vi "Manual_Cool_Heat_V2.vi"(8 "error in":errorcluster, 11 "DataCluster":T1={"Core"={"Current VI Reference"=refnum, "Close Panel on Exit?"=FALSE, "Exit"=FALSE, "Initialized?"=FALSE}, "Connections"={"cDAQ"={"Task"="", "Connected"=FALSE, "Active"=FALSE, "ID"=""}, "Camera"={"Session"="", "Connected"=FALSE, "Active"=FALSE, "Placeholder"=refnum}, "PSU"={"Port"="", "Connected"=FALSE, "Active"=FALSE}, "Arduino"={"Port"="", "Connected"=FALSE, "Active"=FALSE}}, "Data Acquisition"={"Setup"={"Label"="", "Operator"="", "Notes"="", "TempGrad"=0.0, "TargetTemp"=0.0, "Sample Volume"=1.0}, "Camera"={"Image"=refnum, "Save Image"=refnum, "Image Frequency"=20, "Rectangle"={"Left"=0, "Top"=0, "Right"=0, "Bottom"=0, "Rotation"=0.0}, "Calibration"={"Top Left"={"X"=0.0, "Y"=0.0}, "Top Right"={"X"=0.0, "Y"=0.0}, "Bottom Left"={"X"=0.0, "Y"=0.0}, "Bottom Right"={"X"=0.0, "Y"=0.0}, "Fixpoint"={"X"=0.0, "Y"=0.0}, "Scan Area"=0.0, "Fixpoint Area"=0.0, "Well Pixels"=[], "Valid"=FALSE}, "FocusPos"=0, "Display Mapping"=10, "Camera Mode"=10}, "Thermistor"={"Sample Size"=0, "Calibration"={"B0.100"=[], "R25"=[], "c"=[], "State"=[], "V_S"=0.0, "R_S"=0.0}, "Timing Mode"=14713}, "Partition"={"Data"=[], "Cell Label"="", "Cell Color"=0, "Height"=10, "Width"=16, "Grid"=[]}, "Queue"={"Size"=0, "Queue"=refnum}, "Sample Rate"=0, "Active"=FALSE, "Ready"=FALSE, "Graph Mode"=0, "Gradient Buffer"=2}, "Control"={"Sample Rate"=0, "PID gains"={"proportional gain (Kc)"=0.0, "integral time (Ti, min)"=0.0, "derivative time (Td, min)"=0.0}}, "Manual Temp Control"={"TargetTemp"=1.0, "Mode"=0, "Active"=FALSE}} {"Manual Temp Control"."Mode" items=["Cool", "Heat"]; "Manual Temp Control"."TargetTemp" min=-40.0 max=40.0 step=0.5 format="%#_g °C"; "Control"."PID gains"."derivative time (Td, min)" format="%.3f"; "Control"."PID gains"."integral time (Ti, min)" format="%.3f"; "Control"."PID gains"."proportional gain (Kc)" format="%.3f"; "Control"."Sample Rate" min=1 max=20 step=1 format="%.0f Samples/sec"; "Data Acquisition"."Gradient Buffer" min=2 max=30 step=1; "Data Acquisition"."Graph Mode" items=["Thermistor Temperature", "Camera Temperature"]; "Data Acquisition"."Thermistor"."Timing Mode" items=["Automatic"=16097, "High Resolution"=10195, "High Speed"=14712, "Best 50 Hz Rejection"=14713, "Best 60 Hz Rejection"=14714, "Custom"=10137]; "Data Acquisition"."Thermistor"."Calibration"."R_S" min=0.1 max=1000.0 format="%#_g kOhm"; "Data Acquisition"."Thermistor"."Calibration"."V_S" min=5.0 max=48.0 format="%#_g V"; "Data Acquisition"."Thermistor"."Calibration"."R25" min=0.1 max=1000.0 format="%#_g kOhm"; "Data Acquisition"."Thermistor"."Calibration"."B0.100" min=100.0 max=10000.0 format="%#_g K"; "Data Acquisition"."Thermistor"."Sample Size" min=1 max=200; "Data Acquisition"."Sample Rate" min=20 max=240 format="%.0f samples/min"; "Data Acquisition"."Queue"."Size" min=1 max=200; "Data Acquisition"."Camera"."Camera Mode" items=["Temperature Linear", "Signal Linear"]; "Data Acquisition"."Camera"."Display Mapping" items=["Default"=10, "Most Significant Bits"=11, "Full Dynamic"=12, "Downshift"=13, "Given Range"=14, "90% Dynamic"=15, "Given Percent Range"=16]; "Data Acquisition"."Camera"."Calibration"."Fixpoint"."Y" format="%.2f"; "Data Acquisition"."Camera"."Calibration"."Fixpoint"."X" format="%.2f"; "Data Acquisition"."Camera"."Calibration"."Top Left"."Y" format="%.2f"; "Data Acquisition"."Camera"."Calibration"."Top Left"."X" format="%.2f"; "Data Acquisition"."Camera"."Calibration"."Top Right"."Y" format="%.2f"; "Data Acquisition"."Camera"."Calibration"."Top Right"."X" format="%.2f"; "Data Acquisition"."Camera"."Calibration"."Bottom Left"."Y" format="%.2f"; "Data Acquisition"."Camera"."Calibration"."Bottom Left"."X" format="%.2f"; "Data Acquisition"."Camera"."Calibration"."Bottom Right"."Y" format="%.2f"; "Data Acquisition"."Camera"."Calibration"."Bottom Right"."X" format="%.2f"; "Data Acquisition"."Camera"."Rectangle"."Rotation" min=-90.0 max=90.0 step=1.0 format="%.2f"; "Data Acquisition"."Camera"."Rectangle"."Left" scale=0.0..1024.0; "Data Acquisition"."Camera"."Rectangle"."Right" scale=0.0..1024.0; "Data Acquisition"."Camera"."Image Frequency" min=1 max=60 step=1; "Data Acquisition"."Setup"."Sample Volume" min=0.0 max=500.0 format="%#_g µL"; "Data Acquisition"."Setup"."TargetTemp" min=-40.0 max=40.0 step=0.5 format="%#_g °C"; "Data Acquisition"."Setup"."TempGrad" min=-100.0 max=100.0 step=0.1 format="%#_g °C/min"}) -> (0 "error out":errorcluster)   [LabVIEW 2022 SP3]
uses:
  DataCluster.ctl
  <vilib>/userdefined/High Color/IMAQdx.ctl
  <vilib>/vision/Image Controls.llb/IMAQ Image.ctl
  <vilib>/Platform/TimedLoop/XDataNode/timing_clust.ctl
  <vilib>/Platform/TimedLoop/XDataNode/nitl_modes.ctl
  <vilib>/Platform/TimedLoop/XDataNode/wakeup.ctl
  <extravilib>/ChannelInstances/Stream-bool/Read With Abort.vi
  <extravilib>/ChannelInstances/Tag-c(c(ref(LVObjVI()),bool),bool,bool,u32[Cool,Heat])/Write With Abort.vi
  <extravilib>/ChannelInstances/Tag-bool/Write With Abort.vi
  <extravilib>/ChannelInstances/Tag-bool/Read With Abort.vi
  <extravilib>/ChannelInstances/Tag-c(c(ref(LVObjVI()),bool),bool,bool,u32[Cool,Heat])/Read With Abort.vi
  <extravilib>/ChannelInstances/Stream-bool/Write With Abort.vi
  <extravilib>/ChannelInstances/Stream-bool/EndpointRead.vi
  <extravilib>/ChannelInstances/Stream-bool/Endpoint.vi
  <extravilib>/ChannelInstances/Tag-c(c(ref(LVObjVI()),bool),bool,bool,u32[Cool,Heat])/Instantiate.vi
  <extravilib>/ChannelInstances/Tag-bool/Instantiate.vi
  <extravilib>/ChannelInstances/Stream-bool/Instantiate.vi
  <extravilib>/ChannelInstances/Stream-bool/)Channel.vi
  <resource>/ChannelSupport/_ChannelSupport/WaitIfNeeded.vi
  <extravilib>/ChannelInstances/Tag-c(c(ref(LVObjVI()),bool),bool,bool,u32[Cool,Heat])/Endpoint.vi
  <extravilib>/ChannelInstances/Tag-bool/Endpoint.vi
  <extravilib>/ChannelInstances/Tag-bool/EndpointRead.vi
  <extravilib>/ChannelInstances/Tag-c(c(ref(LVObjVI()),bool),bool,bool,u32[Cool,Heat])/EndpointRead.vi
  <vilib>/platform/TimedLoop/XDataNode/XDataNode.xnode
  <vilib>/Platform/TimedLoop/XDataNode/XDNodeRunTimeDep.lvlib
  <extravilib>/ChannelInstances/Tag-bool.lvlib
  <extravilib>/ChannelInstances/Stream-bool.lvlib
  <extravilib>/ChannelInstances/Tag-c(c(ref(LVObjVI()),bool),bool,bool,u32[Cool,Heat]).lvlib
panel:
  in  "Cool/Heat":enum32{"Cool", "Heat"}(ring)
  in  "Start":bool
  in  "OK":bool
  in  "Intensisty":i32(slide)=50 min=0 max=100 step=10 scale=0.0..100.0 scale format="%.0f %%"
  out "Manual":waveform(dbl)[](graph)=[{"t0"=timestamp(0 s since 1904-01-01), "dt"=0.5, "Y"=[-0.5459297948238789, -0.5384662523625495, -0.5305055716687722, -0.5227516337304128, -0.5152151485633342, -0.5074594731778411, -0.5000110550794236, -0.49229613528221505, -0.48455544270581347, -0.47704875214651904, -0.4694184221817747, -0.4617297562684411, -0.4542538363910736, -0.44666324774779786, -0.43914993037163397, -0.4315969934450372, -0.42413652957329057, -0.41648702187743, -0.4090503718449979, -0.40158637492342547, -0.3941665018638969, -0.38661414017374235, -0.3792972035366138, -0.37178469009330656, -0.3640722423599955, -0.3568479440776631, -0.3495051306403334, -0.3421642645601655, -0.33493653098477, -0.3275193397439705, -0.32018295336060504, -0.3128894600430486, -0.3055440591103306, -0.29873448073929, -0.29143683883588484, -0.2843423086450982, -0.2772355209388995, -0.27008916517709947, -0.26279625635638254, -0.2557072429162988, -0.24884447893036513, -0.2418962610460262, -0.23471006933283486, -0.22766777081987025, -0.22069024864064335, -0.21390317409486895, -0.20710909597313554, -0.20017922598796378, -0.19328186072145903, -0.18648965958030286, -0.17982101574808698, -0.17308125272085514, -0.16650153019624944, -0.15972005812583243, -0.15288052381799008, -0.14672994680516058, -0.14007374846858675, -0.1336178193214643, -0.12705690492929214, -0.12060549031730709, -0.11444511771368156, -0.10804984536035589, -0.10172786836292154, -0.09532872836465985, -0.08927381125350682, -0.08296971036909855, -0.07689207711853907, -0.07078036829076739, -0.06468688490901309, -0.058868939175738766, -0.05270999822746214, -0.04685361027102993, -0.04104637566433278]}, {"t0"=timestamp(0 s since 1904-01-01), "dt"=0.5, "Y"=[-30.0, -30.0, -30.0, -30.0, -30.0, -30.0, -30.0, -30.0, -30.0, -30.0, -30.0, -30.0, -30.0, -30.0, -30.0, -30.0, -30.0, -30.0, -30.0, -30.0, -30.0, -30.0, -30.0, -30.0, -30.0, -30.0, -30.0, -30.0, -30.0, -30.0, -30.0, -30.0, -30.0, -30.0, -30.0, -30.0, -30.0, -30.0, -30.0, -30.0, -30.0, -30.0, -30.0, -30.0, -30.0, -30.0, -30.0, -30.0, -30.0, -30.0, -30.0, -30.0, -30.0, -30.0, -30.0, -30.0, -30.0, -30.0, -30.0, -30.0, -30.0, -30.0, -30.0, -30.0, -30.0, -30.0, -30.0, -30.0, -30.0, -30.0, -30.0, -30.0, -30.0]}]
  out "Status":string="System ready"
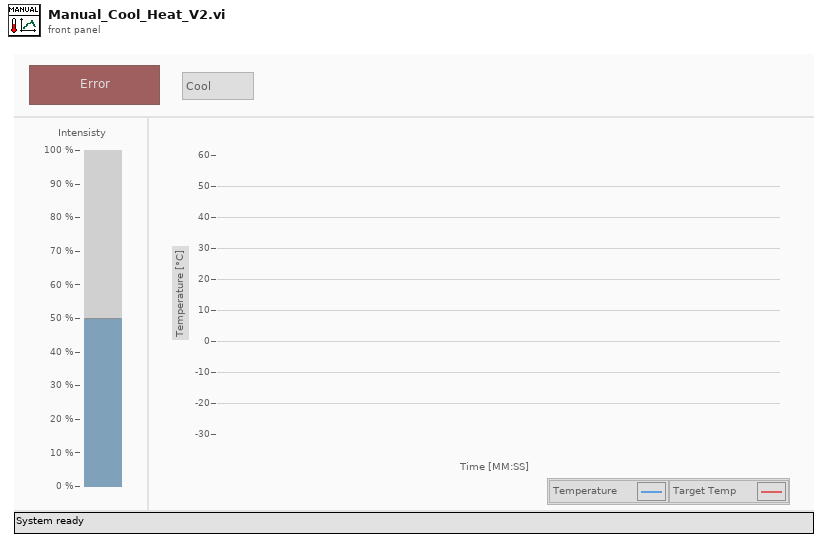
[diagram p1: front panel]
types:
  T1 = typedef "DataCluster.ctl" = cluster{"Core":cluster{"Current VI Reference":refnum<vi>, "Close Panel on Exit?":bool, "Exit":bool, "Initialized?":bool}, "Connections":cluster{"cDAQ":cluster{"Task":refnum<k21>, "Connected":bool, "Active":bool, "ID":string}, "Camera":cluster{"Session":T2, "Connected":bool, "Active":bool, "Placeholder":T3}, "PSU":cluster{"Port":refnum<visa-resource-name>, "Connected":bool, "Active":bool}, "Arduino":cluster{"Port":refnum<visa-resource-name>, "Connected":bool, "Active":bool}}, "Data Acquisition":cluster{"Setup":cluster{"Label":string, "Operator":string, "Notes":string, "TempGrad":dbl, "TargetTemp":dbl, "Sample Volume":dbl}, "Camera":cluster{"Image":T3, "Save Image":T3, "Image Frequency":i32, "Rectangle":T4, "Calibration":cluster{"Top Left":T5, "Top Right":T5, "Bottom Left":T5, "Bottom Right":T5, "Fixpoint":T5, "Scan Area":dbl, "Fixpoint Area":dbl, "Well Pixels":cluster{"X":i32, "Y":i32}[][], "Valid":bool}, "FocusPos":u32, "Display Mapping":u32, "Camera Mode":u32}, "Thermistor":cluster{"Sample Size":i32, "Calibration":cluster{"B0.100":dbl[], "R25":dbl[], "c":dbl[][], "State":bool[], "V_S":dbl, "R_S":dbl}, "Timing Mode":i32}, "Partition":cluster{"Data":string[][], "Cell Label":string, "Cell Color":u32, "Height":i32, "Width":i32, "Grid":string[][]}, "Queue":cluster{"Size":i32, "Queue":refnum<queue>}, "Sample Rate":i32, "Active":bool, "Ready":bool, "Graph Mode":u16, "Gradient Buffer":i32}, "Control":cluster{"Sample Rate":i32, "PID gains":cluster{"proportional gain (Kc)":dbl, "integral time (Ti, min)":dbl, "derivative time (Td, min)":dbl}}, "Manual Temp Control":cluster{"TargetTemp":dbl, "Mode":u16, "Active":bool}}
  T2 = typedef "IMAQdx.ctl" = refnum<k21>
  T3 = typedef "IMAQ Image.ctl" = refnum<image>
  T4 = typedef "IMAQ Rectangle" = cluster{"Left":i32, "Top":i32, "Right":i32, "Bottom":i32, "Rotation":dbl}
  T5 = typedef "IMAQ Point" = cluster{"X":sgl, "Y":sgl}
  T6 = enum8{"Enabled", "Disabled", "Disabled and Grayed Out"}
  T7 = enum32{"Invalid", "Standard", "Closed", "Hidden", "Minimized", "Maximized"}
  T8 = enum32{"invalid app kind", "Development System", "Run Time System", "Student Edition", "Embedded LabVIEW", "Evaluation", "Custom"}
  T9 = cluster{"Core":cluster{"Current VI Reference":refnum<vi>, "Close Panel on Exit?":bool}, "Active":bool, "Ready":bool, "Cool/Heat":enum32{"Cool", "Heat"}}
  T10 = cluster{"Current VI Reference":refnum<vi>, "Close Panel on Exit?":bool}
  T11 = typedef "Tag-bool.lvlib/))Channel.ctl" = refnum<queue>
  T12 = typedef "Tag-c(c(ref(LVObjVI()),bool),bool,bool,u32[Cool,Heat]).lvlib/))Channel.ctl" = refnum<queue>
  T13 = typedef "XDNodeRunTimeDep.lvlib/timing_clust.ctl" = cluster{"Expected End [f-1]":u64, "Actual End [f-1]":u64, "Finished Late? [f-1]":bool, "Expected End [i-1]":u64, "Actual End [i-1]":u64, "Finished Late? [i-1]":bool, "Expected Start [i]":u64, "Actual Start [i]":u64, "Expected Start [f]":u64, "Actual Start [f]":u64, "Source Name":string, "Structure Name":string, "Period":i64, "Deadline":i64, "Offset":i64, "Start":i64, "Priority":i32, "Timeout":i32, "Mode":T14, "Wakeup Reason":T15, "Error":errorcluster, "Source Type":string, "Secondary Source Type":string, "Global End Time":u64, "Global Start Time":u64, "Frame Duration":u64, "Iteration Duration":u64, "Assigned CPU":i32, "I/O Scan Engine Mode":u32}
  T14 = typedef "XDNodeRunTimeDep.lvlib/nitl_modes.ctl" = enum32{"No Change", "Process missed periods, maintain original phase", "Discard missed periods, maintain original phase", "Process missed periods, ignore original phase", "Discard missed periods, ignore original phase"}
  T15 = typedef "XDNodeRunTimeDep.lvlib/wakeup.ctl" = enum32{"Normal", "Aborted", "Asynchronous wakeup", "Timing source error", "Timed loop error", "Timeout"}
  T16 = typedef "Stream-bool.lvlib/)Channel.ctl" = refnum<queue>
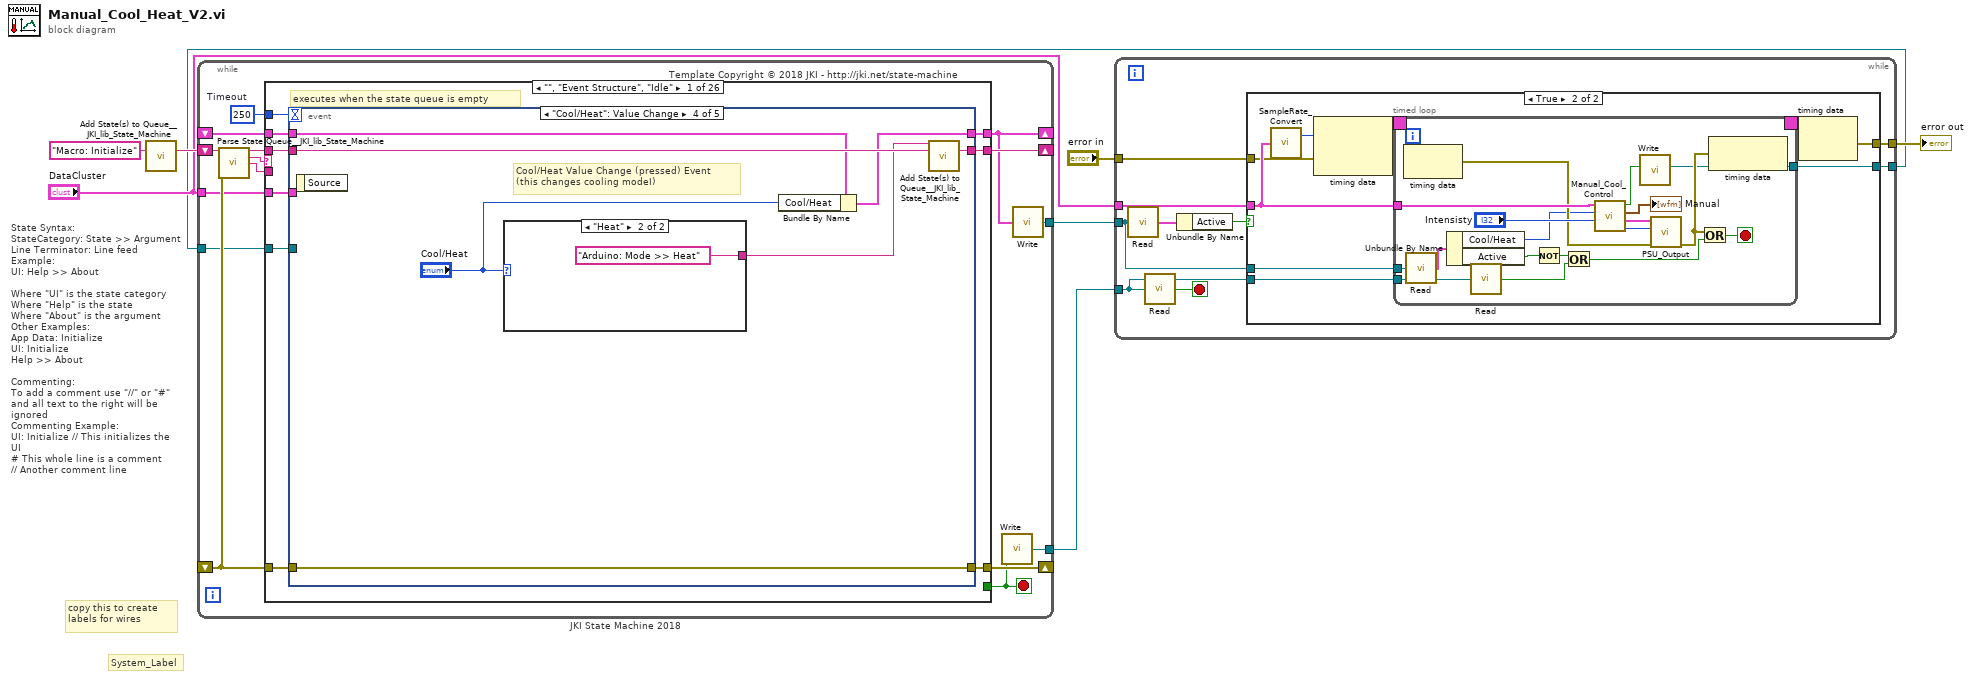
[diagram p0: block diagram]
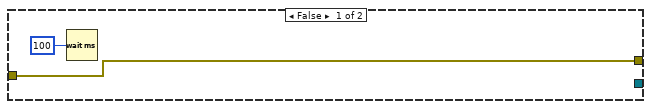
[diagram p2: hidden frame]
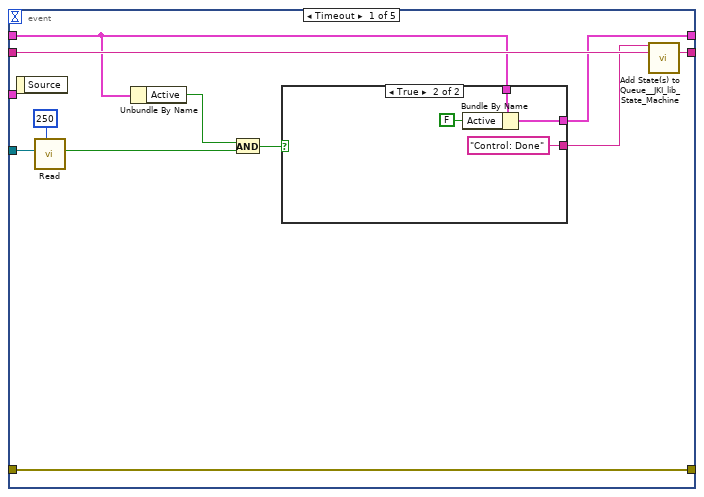
[diagram p3: hidden frame]
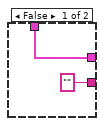
[diagram p4: hidden frame]
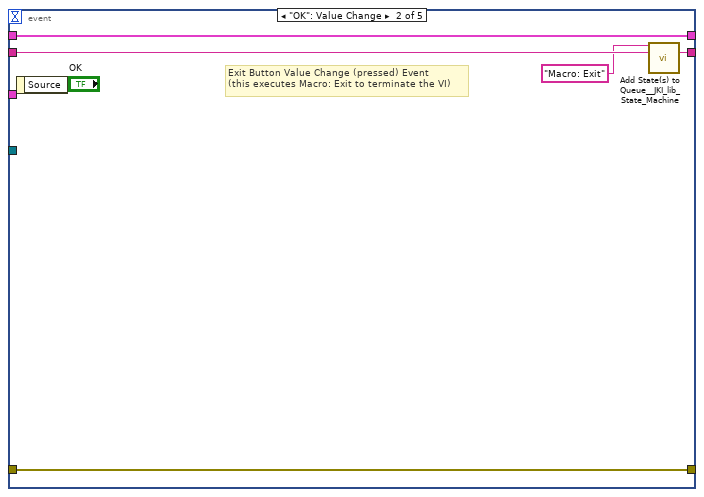
[diagram p5: hidden frame]
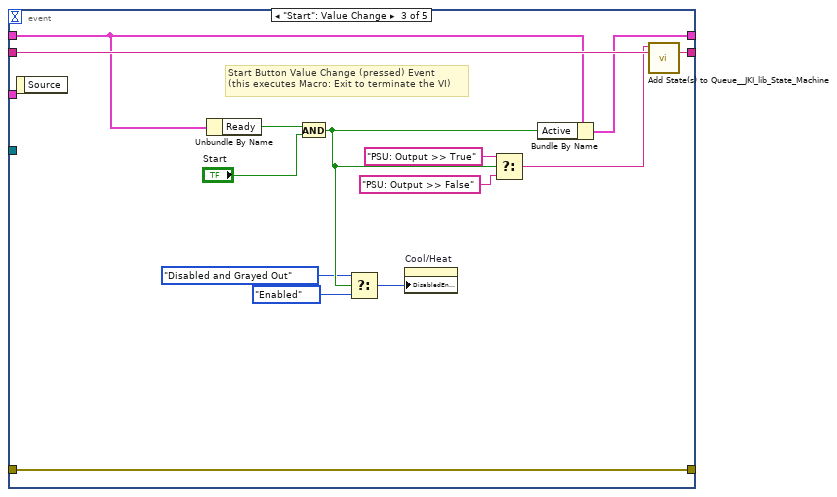
[diagram p6: hidden frame]
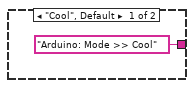
[diagram p7: hidden frame]
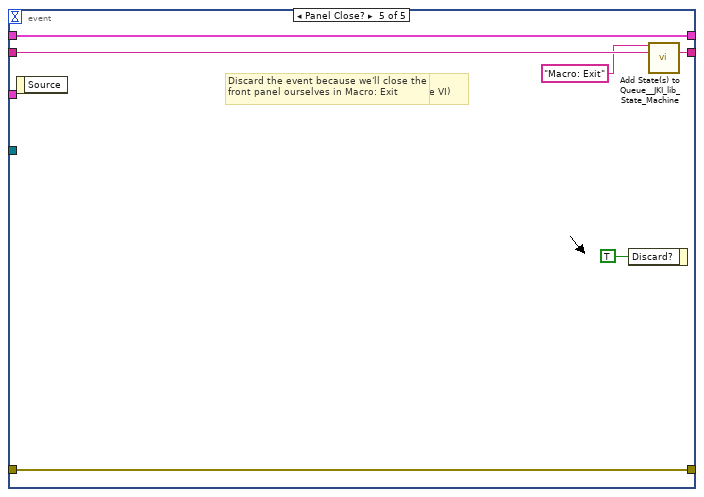
[diagram p8: hidden frame]
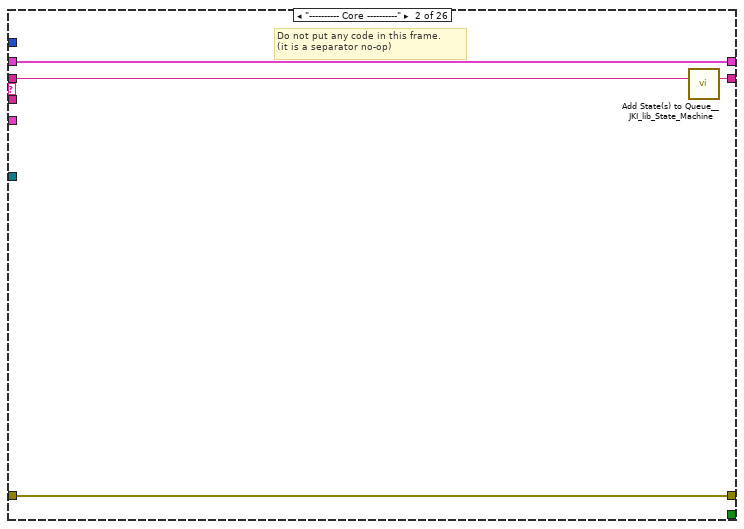
[diagram p9: hidden frame]
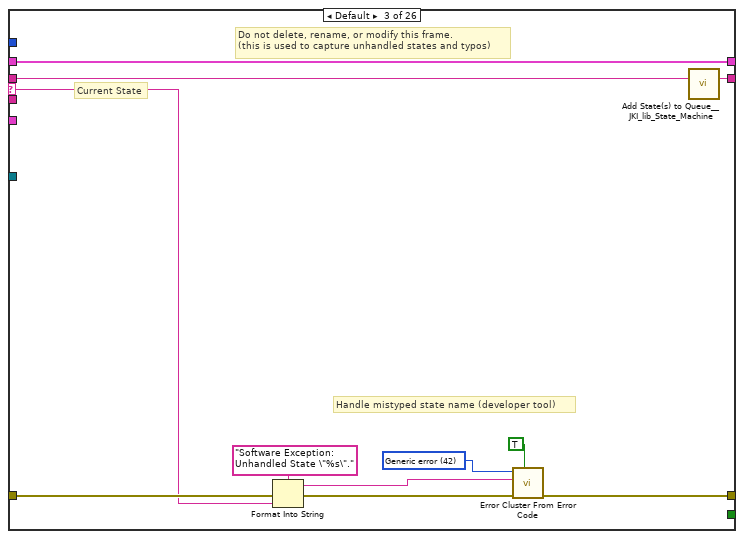
[diagram p10: hidden frame]
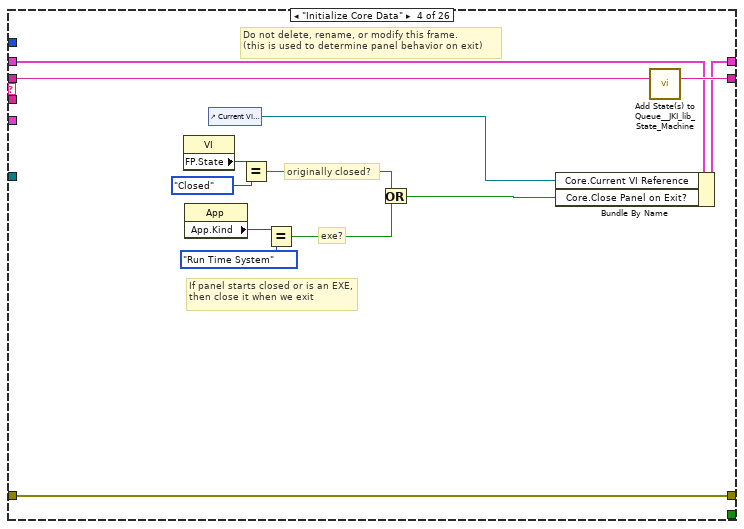
[diagram p11: hidden frame]
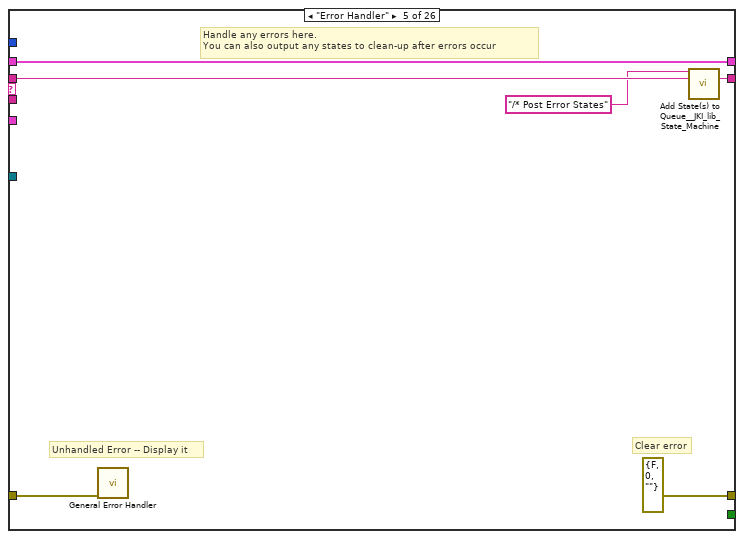
[diagram p12: hidden frame]
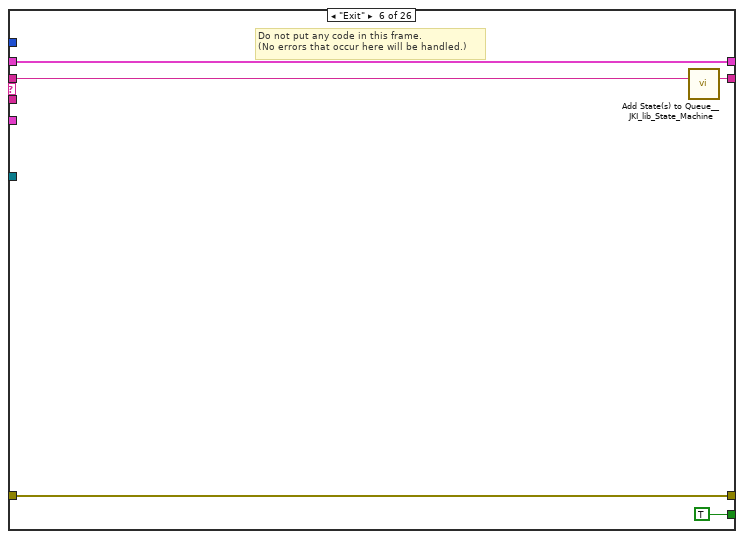
[diagram p13: hidden frame]
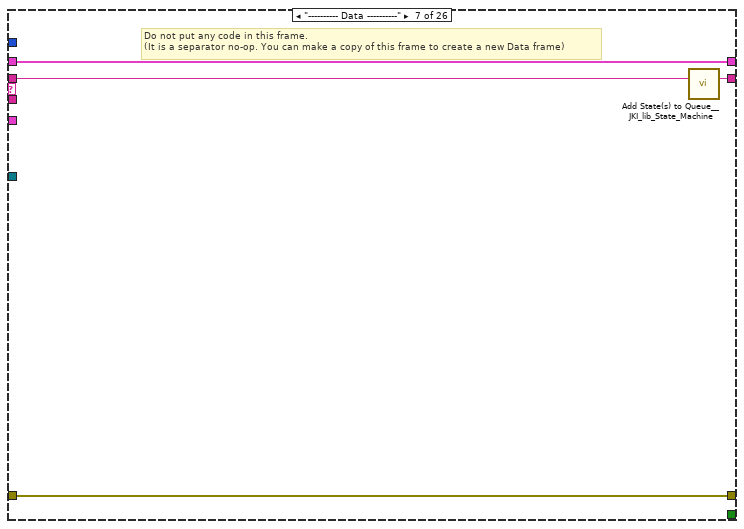
[diagram p14: hidden frame]
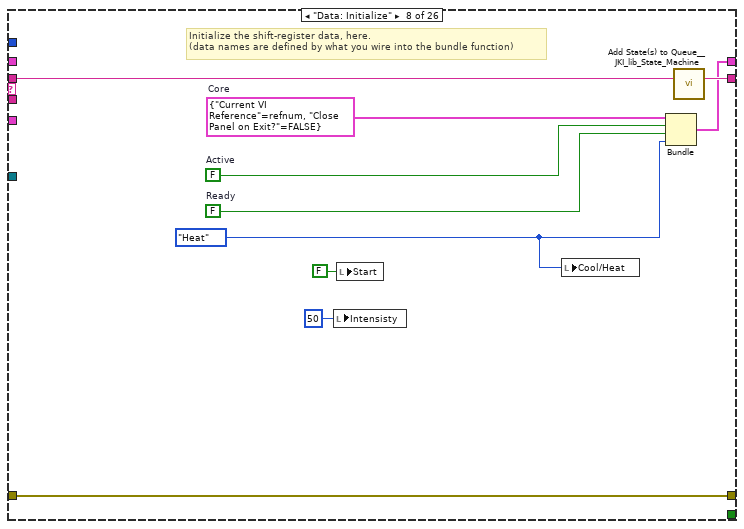
[diagram p15: hidden frame]
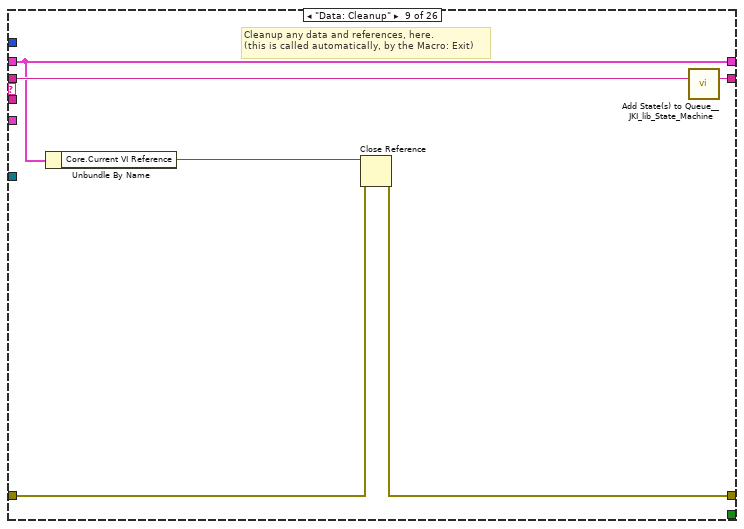
[diagram p16: hidden frame]
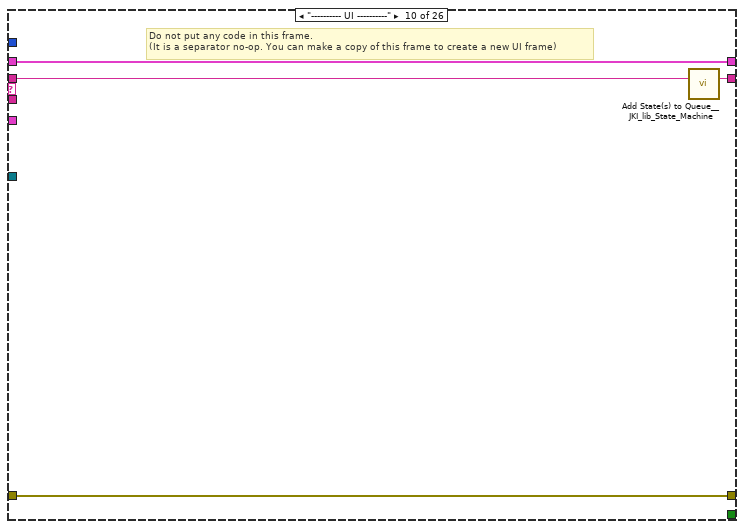
[diagram p17: hidden frame]
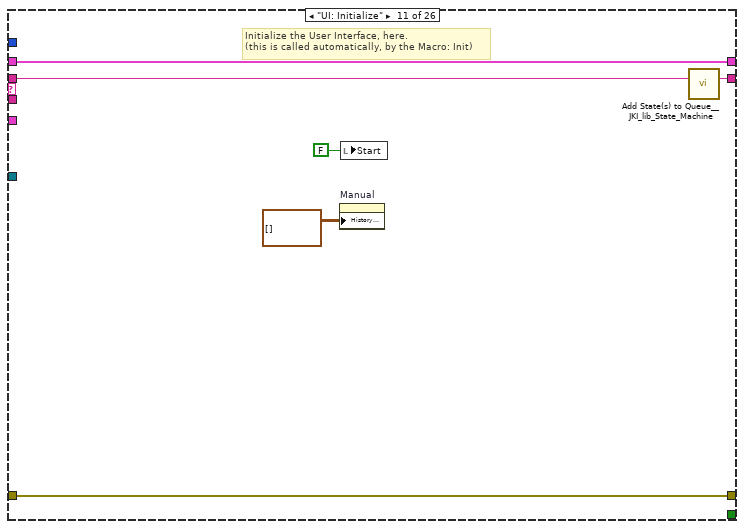
[diagram p18: hidden frame]
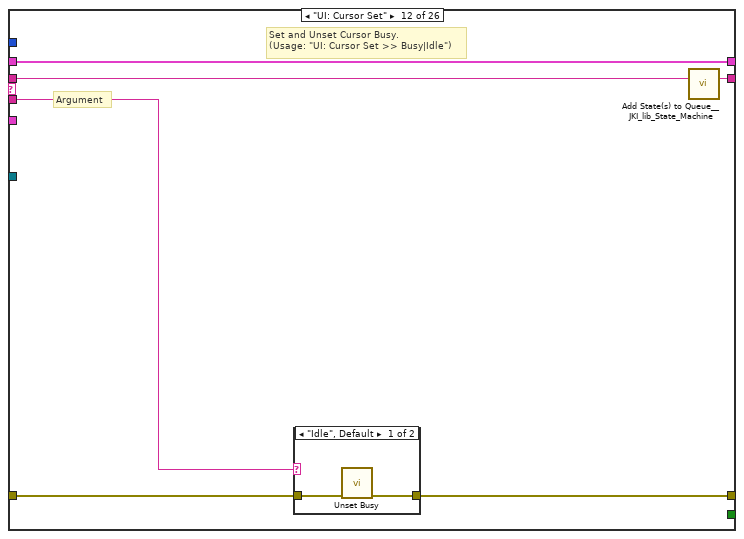
[diagram p19: hidden frame]
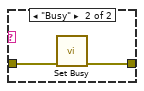
[diagram p20: hidden frame]
diagram:
  # "State Syntax:\nStateCategory: State >> Argument\nLine Terminator: Line feed\nExample:\nUI: Help >> About\n\nWhere \"UI\" is the state category\nWhere \"Help\" is the state\nWhere \"About\" is the argument\nOther Examples:\nApp Data: Initialize\nUI: Initialize\nHelp >> About\n\nCommenting:\nTo add a comment use \"//\" or \"#\" and all text to the right will be ignored\nCommenting Example:\nUI: Initialize // This initializes the UI\n# This whole line is a comment\n// Another comment line"
  # "copy this to create labels for wires"
  # "System_Label"
  n1 = call <vilib>:"Add State(s) to Queue__JKI_lib_State_Machine.vi"("State(s) in (\"\")"="Macro: Initialize") -> ("States Out"=w8:string)  [unwired: 14 in]
  n2 = while "JKI State Machine 2018" {
    shift-right: [w16] -> _
    shift-left: _ -> [w15]
    shift-right: [w19] -> _
    shift-left: _ -> [w13]
    shift-right: [w18] -> _
    shift-left: w8 -> [w20]
    tunnel: "DataCluster" -> [w12]
    tunnel: w3 -> [w11]
    tunnel: [w10] -> w2
    tunnel: [w9] -> w1
    stop <- w17 stop-if-true
    w14 = 250  # Timeout
    # "Template Copyright © 2018 JKI - http://jki.net/state-machine"
    n3 = call <vilib>:"Parse State Queue__JKI_lib_State_Machine.vi"("State Queue"=w20, "Error In (no error)"=w13) -> ("Remaining States"=w22:string, "Current State"=w23:string, "Arguments"=w21:string)  [unwired: 11 in]
    n4 = case shown="\"\", \"Event Structure\", \"Idle\"" w23 {
      selector: w23 -> [_ _ w88 _ _ _ _ _ _ _ _ _ _ _ _ _ _ _ _ _ _ _ _ _ _ _]
      tunnel: w22 -> [w32 w87 w92 w111 w117 w122 w126 w136 w142 w146 w152 w158 w167 w174 w243 w248 w258 w262 w278 w286 w295 w316 w323 w327 w335 w346]
      tunnel: w21 -> [_ _ _ _ _ _ _ _ _ _ _ w153 w163 w168 _ _ _ _ _ _ _ _ _ _ w330 w342]
      tunnel: w15 -> [w30 w84 w90 w104 w114 w120 w123 _ w137 w143 w150 w156 w165 w170 w240 w245 w255 w259 w275 w284 w293 w314 w319 w324 w333 w344]
      tunnel: [w29 w85 w94 w108 errorcluster {"status"=FALSE, "code"=0, "source"=""} ("error out") w119 w124 w133 w138 w144 w149 w154 w164 w171 w241 w246 w256 w260 w276 w283 w292 w313 w321 w325 w328 w341] -> w19
      tunnel: w13 -> [w28 w85 w93 w108 w113 w119 w124 w133 w139 w144 w149 w155 w164 w172 w241 w246 w256 w260 w276 w283 w292 w313 w321 w325 w329 w341]
      tunnel: [w31 w86 w91 w110 w116 w121 w125 w135 w141 w145 w151 w157 w166 w173 w242 w247 w257 w261 w277 w285 w294 w315 w322 w326 w334 w345] -> w18
      tunnel: [_ _ _ _ _ TRUE _ _ _ _ _ _ _ _ _ _ _ _ _ _ _ _ _ _ _ _] -> w17
      tunnel: [w27 w84 w90 w109 w114 w120 w123 w134 w137 w143 w150 w156 w165 w170 w240 w245 w255 w259 w267 w284 w293 w314 w320 w324 w333 w344] -> w16
      tunnel: w14 -> [w26 _ _ _ _ _ _ _ _ _ _ _ _ _ _ _ _ _ _ _ _ _ _ _ _ _]
      tunnel: w12 -> [w25 _ _ _ _ _ _ _ _ _ _ _ _ _ _ _ _ _ w274 _ _ w310 _ _ w331 w343]
      tunnel: w11 -> [w24 _ _ _ _ _ _ _ _ _ _ _ _ _ _ _ _ _ _ _ _ _ _ _ _ _]
      frame "", "Event Structure", "Idle" {
        # "executes when the state queue is empty"
        n5 = event shown="[3] \"Cool/Heat\": Value Change" {
          selector: _ -> [_ _ _ _ _]
          dyn-events: _ -> [_ _ _ _ _]
          timeout: w26 -> [_ _ _ _ _]
          tunnel: w32 -> [w43 w54 w68 w75 w83]
          tunnel: [w42 w53 w67 w74 w82] -> w31
          tunnel: w30 -> [w39 w51 w61 w72 w80]
          tunnel: [w41 w52 w66 w73 w81] -> w29
          tunnel: w28 -> [w41 w52 w66 w73 w81]
          tunnel: [w36 w51 w62 w70 w80] -> w27
          tunnel: w25 -> [_ _ _ _ _]
          tunnel: w24 -> [w40 _ _ _ _]
          event Timeout {
            n6 = event-data() -> ()  [unwired: 1 in, 1 out]
            n7 = call <extravilib>:"Read.vi"("timeout in ms (-1)"=250, "channel"=w40) -> ("element"=w37:bool)  [unwired: 5 in, 4 out]
            n8 = Unbundle By Name(w39) -> ("Active"=w38:bool)
            n9 = And(x=w38, y=w37) -> (x .and. y?=w34:bool)
            n10 = case shown="True" w34 {
              tunnel: w39 -> [w45 w49]
              tunnel: [w45 w48] -> w36
              tunnel: ["" "Control: Done"] -> w33
              frame False {
              }
              frame True {
                n11 = Bundle By Name(cluster=w49, "Active"=FALSE) -> (w48:T9)
              }
            }
            n12 = call <vilib>:"Add State(s) to Queue__JKI_lib_State_Machine.vi"("State(s) in Front (\"\")"=w33, "State(s) in (\"\")"=w43) -> ("States Out"=w42:string)  [unwired: 13 in]
          }
          event "OK": Value Change {
            # "Exit Button Value Change (pressed) Event\n(this executes Macro: Exit to terminate the VI)"
            n13 = event-data() -> ()  [unwired: 1 in, 1 out]
            n14 = call <vilib>:"Add State(s) to Queue__JKI_lib_State_Machine.vi"("State(s) in Front (\"\")"="Macro: Exit", "State(s) in (\"\")"=w54) -> ("States Out"=w53:string)  [unwired: 13 in]
          }
          event "Start": Value Change {
            # "Start Button Value Change (pressed) Event\n(this executes Macro: Exit to terminate the VI)"
            n15 = event-data() -> ()  [unwired: 1 in, 1 out]
            n16 = Unbundle By Name(w61) -> ("Ready"=w60:bool)
            n17 = And(x=w60, y="Start") -> (x .and. y?=w58:bool)
            n18 = Select(t=T6."Disabled and Grayed Out" ("Disabled"), s=w58, f=T6."Enabled" ("Disabled")) -> (s? t:f=w57:T6)
            n19 = property on="Cool/Heat" class="Enum (strict)"("DisabledEnum"=w57) -> ()  [unwired: 2 in, 2 out]
            n20 = Select(t="PSU: Output >> True", s=w58, f="PSU: Output >> False") -> (s? t:f=w63:string)
            n21 = Bundle By Name(cluster=w61, "Active"=w58) -> (w62:T9)
            n22 = call <vilib>:"Add State(s) to Queue__JKI_lib_State_Machine.vi"("State(s) in Front (\"\")"=w63, "State(s) in (\"\")"=w68) -> ("States Out"=w67:string)  [unwired: 13 in]
          }
          event "Cool/Heat": Value Change {
            # "Cool/Heat Value Change (pressed) Event\n(this changes cooling modeI)"
            n23 = event-data() -> ()  [unwired: 1 in, 1 out]
            n24 = case shown="\"Heat\"" "Cool/Heat" {
              tunnel: ["Arduino: Mode >> Cool" "Arduino: Mode >> Heat"] -> w71
              frame "Cool", Default {
              }
              frame "Heat" {
              }
            }
            n25 = Bundle By Name(cluster=w72, "Cool/Heat"="Cool/Heat") -> (w70:T9)
            n26 = call <vilib>:"Add State(s) to Queue__JKI_lib_State_Machine.vi"("State(s) in Front (\"\")"=w71, "State(s) in (\"\")"=w75) -> ("States Out"=w74:string)  [unwired: 13 in]
          }
          event Panel Close? {
            # "Discard the event because we'll close the front panel ourselves in Macro: Exit"
            # "Close Panel button (pressed) Event\n(this executes Macro: Exit to terminate the VI)"
            n27 = event-data() -> ()  [unwired: 1 in, 1 out]
            n28 = event-data("Discard?"=TRUE) -> ()  [unwired: 1 in, 1 out]
            n29 = call <vilib>:"Add State(s) to Queue__JKI_lib_State_Machine.vi"("State(s) in Front (\"\")"="Macro: Exit", "State(s) in (\"\")"=w83) -> ("States Out"=w82:string)  [unwired: 13 in]
          }
        }
      }
      frame "---------- Core ----------" {
        # "Do not put any code in this frame.\n(it is a separator no-op)"
        n30 = call <vilib>:"Add State(s) to Queue__JKI_lib_State_Machine.vi"("State(s) in (\"\")"=w87) -> ("States Out"=w86:string)  [unwired: 14 in]
      }
      frame Default {
        w97 = 42 items=["No error", "Argument error", "Memory is full", "Out of zone", "End of file", "File already open", "Generic file I/O error", "File not found", "File permission error", "Disk is full", "Duplicate path", "Too many files open", "System feature not enabled", "Resource file not found", "Cannot add resource", "Resource not found", "Image not found", "Image memory error", "Pen does not exist", "Config type invalid", "Config token not found", "Config parse error", "Config memory error", "Bad external code format", "Bad external code offset", "External code not present", "Null window", "Destroy window error", "Null menu", "Print aborted", "Bad print record", "Print driver error", "Windows error during printing", "Memory error during printing", "Print dialog error", "Generic print error", "Invalid device refnum", "Device not found", "Device parameter error", "Device unit error", "Cannot open device", "Device call aborted", "Generic error", "Cancelled by user", "Object ID too low", "Object ID too high", "Object not in heap", "Unknown heap", "Unknown object (invalid DefProc)", "Unknown object (DefProc not in table)", "Message out of range", "Invalid (null) method", "Unknown message", "Manager call not supported", "Bad address", "Network operation in progress", "Network operation timed out", "Connection is busy", "Network attribute not supported", "Network error", "Address in use", "System out of memory", "Connection aborted", "Connection refused", "Not connected", "Already connected", "Connection closed", "Initialization error (interapplication manager)", "Bad occurrence", "Wait on unbound occurrence handler", "Occurrence queue overflow", "Datalog type conflict", "Unused", "Unrecognized type (interapplication manager)", "Memory corrupt", "Failed to make temporary DLL", "Old CIN version", "Drag socket not found", "Failed to load drop-object", "Failed to register OLE object", "Failed to release OLE object", "Format specifier type mismatch", "Unknown format specifier", "Too few format specifiers", "Too many format specifiers", "Scan failed", "Newer CIN version", "Error converting to variant", "Runtime menu error", "Password tampered", "Variant attribute not found", "Incompatible variant data type", "Event data is not available", "Event Store is not present", "Occurrence is not found", "Event Queue is not created", "Event info is not available", "Refnum passed is NULL", "Error retrieving Class GUID", "Error retrieving CoClass GUID", "Error retrieving TypeLib GUID.", "Bad built application magic bytes.", "Specific driver is different from the specific driver associated with the Logical Name.", "There is no session opened to the class driver.", "Max Error", "MAX - Error with config objects", "MAX - Error loading configuration", "MAX - Group not supported"]
        # "Current State"
        # "Do not delete, rename, or modify this frame.\n(this is used to capture unhandled states and typos)"
        # "Handle mistyped state name (developer tool)"
        n31 = Format Into String(format string="Software Exception: Unhandled State \"%s\"." ("message"), error in=w93, w88) -> (resulting string=w96:string, error out=w95:errorcluster)  [unwired: 1 in]
        n32 = call <vilib>:"Error Cluster From Error Code.vi"("show call chain? (False)"=TRUE, "error in (no error)"=w95, "error message (\"\")"=w96, "error code (0)"=w97) -> ("error out"=w94:errorcluster)  [unwired: 5 in]
        n33 = call <vilib>:"Add State(s) to Queue__JKI_lib_State_Machine.vi"("State(s) in (\"\")"=w92) -> ("States Out"=w91:string)  [unwired: 14 in]
      }
      frame "Initialize Core Data" {
        # "Do not delete, rename, or modify this frame.\n(this is used to determine panel behavior on exit)"
        # "originally closed?"
        # "exe?"
        # "If panel starts closed or is an EXE, then close it when we exit"
        n34 = property class="VI"() -> ("FP.State"=w101:T7)  [unwired: 2 in, 2 out]
        n35 = property class="App"() -> ("App.Kind"=w107:T8)  [unwired: 2 in, 2 out]
        n36 = control-ref of="Current VI Reference"() -> (w102:refnum<vi>)
        n37 = Equal?(x=w101, y=T7."Closed" ("Front Panel Window:State")) -> (x = y?=w99:bool)
        n38 = Equal?(x=w107, y=T8."Run Time System" ("Application:Kind")) -> (x = y?=w105:bool)
        n39 = Or(x=w99, y=w105) -> (x .or. y?=w103:bool)
        n40 = Bundle By Name(cluster=w104, "Core.Current VI Reference"=w102, "Core.Close Panel on Exit?"=w103) -> (w109:T9)
        n41 = call <vilib>:"Add State(s) to Queue__JKI_lib_State_Machine.vi"("State(s) in (\"\")"=w111) -> ("States Out"=w110:string)  [unwired: 14 in]
      }
      frame "Error Handler" {
        # "Unhandled Error -- Display it"
        # "Handle any errors here.\nYou can also output any states to clean-up after errors occur"
        # "Clear error"
        n42 = call <vilib>:"General Error Handler.vi"("error in (no error)"=w113) -> ()  [unwired: 10 in, 5 out]
        n43 = call <vilib>:"Add State(s) to Queue__JKI_lib_State_Machine.vi"("State(s) in Front (\"\")"="/* Post Error States", "State(s) in (\"\")"=w117) -> ("States Out"=w116:string)  [unwired: 13 in]
      }
      frame "Exit" {
        # "Do not put any code in this frame.\n(No errors that occur here will be handled.)"
        n44 = call <vilib>:"Add State(s) to Queue__JKI_lib_State_Machine.vi"("State(s) in (\"\")"=w122) -> ("States Out"=w121:string)  [unwired: 14 in]
      }
      frame "---------- Data ----------" {
        # "Do not put any code in this frame.\n(It is a separator no-op. You can make a copy of this frame to create a new Data frame)"
        n45 = call <vilib>:"Add State(s) to Queue__JKI_lib_State_Machine.vi"("State(s) in (\"\")"=w126) -> ("States Out"=w125:string)  [unwired: 14 in]
      }
      frame "Data: Initialize" {
        w127 = enum32{"Cool", "Heat"}."Heat" ("Cool/Heat")
        w130 = FALSE  # Ready
        w131 = T10 {"Current VI Reference"=refnum, "Close Panel on Exit?"=FALSE}  # Core
        w132 = FALSE  # Active
        # "Initialize the shift-register data, here.\n(data names are defined by what you wire into the bundle function)"
        n46 = local write "Intensisty"(50 ("Intensisty")) -> ()
        n47 = local write "Start"(FALSE ("Key Focus")) -> ()
        n48 = local write "Cool/Heat"(w127) -> ()
        n49 = Bundle("Core"=w131, "Active"=w132, "Ready"=w130, "Cool/Heat"=w127) -> (w134:T9)  [unwired: 1 in]
        n50 = call <vilib>:"Add State(s) to Queue__JKI_lib_State_Machine.vi"("State(s) in (\"\")"=w136) -> ("States Out"=w135:string)  [unwired: 14 in]
      }
      frame "Data: Cleanup" {
        # "Cleanup any data and references, here.\n(this is called automatically, by the Macro: Exit)"
        n51 = Unbundle By Name(w137) -> ("Core.Current VI Reference"=w140:refnum<vi>)
        n52 = Close Reference(reference=w140, error in (no error)=w139) -> (error out=w138:errorcluster)
        n53 = call <vilib>:"Add State(s) to Queue__JKI_lib_State_Machine.vi"("State(s) in (\"\")"=w142) -> ("States Out"=w141:string)  [unwired: 14 in]
      }
      frame "---------- UI ----------" {
        # "Do not put any code in this frame.\n(It is a separator no-op. You can make a copy of this frame to create a new UI frame)"
        n54 = call <vilib>:"Add State(s) to Queue__JKI_lib_State_Machine.vi"("State(s) in (\"\")"=w146) -> ("States Out"=w145:string)  [unwired: 14 in]
      }
      frame "UI: Initialize" {
        # "Initialize the User Interface, here.\n(this is called automatically, by the Macro: Init)"
        n55 = property on="Manual" class="WFChart (strict)"("History Data"=waveform(dbl)[][] []) -> ()  [unwired: 2 in, 2 out]
        n56 = local write "Start"(FALSE ("Accept Values")) -> ()
        n57 = call <vilib>:"Add State(s) to Queue__JKI_lib_State_Machine.vi"("State(s) in (\"\")"=w152) -> ("States Out"=w151:string)  [unwired: 14 in]
      }
      frame "UI: Cursor Set" {
        # "Argument"
        # "Set and Unset Cursor Busy.\n(Usage: \"UI: Cursor Set >> Busy|Idle\")"
        n58 = case shown="\"Idle\", Default" w153 {
          tunnel: w155 -> [w160 w162]
          tunnel: [w159 w161] -> w154
          frame "Idle", Default {
            n59 = call <vilib>:"Unset Busy.vi"("error in (no error)"=w160) -> ("error out"=w159:errorcluster)  [unwired: 10 in]
          }
          frame "Busy" {
            n60 = call <vilib>:"Set Busy.vi"("error in (no error)"=w162) -> ("error out"=w161:errorcluster)  [unwired: 9 in, 1 out]
          }
        }
        n61 = call <vilib>:"Add State(s) to Queue__JKI_lib_State_Machine.vi"("State(s) in (\"\")"=w158) -> ("States Out"=w157:string)  [unwired: 14 in]
      }
      frame "UI: Status" {
        # "Argument"
        # "Set and Unset Cursor Busy.\n(Usage: \"UI: Cursor Set >> Busy|Idle\")"
        n62 = call <vilib>:"Add State(s) to Queue__JKI_lib_State_Machine.vi"("State(s) in (\"\")"=w167) -> ("States Out"=w166:string)  [unwired: 14 in]
        "Status" <- w163
      }
      frame "UI: Front Panel State" {
        # "Argument"
        # "Set Front Panel Open or Closed\n(Usage: \"UI: Front Panel State >> Open|Close\")"
        n63 = Unbundle By Name(w170) -> ("Core.Current VI Reference"=w169:refnum<vi>)
        n64 = case shown="\"Minimize\", \"Minimized\"" w168 {
          tunnel: w172 -> [w180 w195 w206 w219 w232]
          tunnel: [w182 w196 w208 w221 w234] -> w171
          tunnel: w169 -> [w181 w193 w207 w220 w233]
          frame "Open", "Standard", Default {
            w175 = T7."Standard" ("State")
            n65 = property class="VI"(reference=w181, error in=w180) -> (reference out=w178:refnum<vi>, error out=w179:errorcluster, "FP.State"=w177:T7)
            n66 = Not Equal?(x=w177, y=w175) -> (x != y?=w176:bool)
            n67 = case shown="True" w176 {
              tunnel: [w186 w188] -> w182
              tunnel: w179 -> [w185 w188]
              tunnel: w178 -> [w184 _]
              tunnel: w175 -> [w183 _]
              frame True {
                n68 = invoke class="VI" method="FP.Open"(reference=w184, error in=w185, "Activate"=TRUE, "State"=w183) -> (error out=w186:errorcluster)  [unwired: 1 in, 4 out]
              }
              frame False {
              }
            }
          }
          frame "Close", "Closed" {
            n69 = property class="VI"(reference=w193, error in=w195) -> (reference out=w192:refnum<vi>, error out=w194:errorcluster, "FP.State"=w190:T7)
            n70 = Not Equal?(x=w190, y=T7."Closed" ("Front Panel Window:State")) -> (x != y?=w189:bool)
            n71 = case shown="True" w189 {
              tunnel: [w197 w200] -> w196
              tunnel: w194 -> [w197 w199]
              tunnel: w192 -> [_ w198]
              frame False {
              }
              frame True {
                n72 = invoke class="VI" method="FP.Close"(reference=w198, error in=w199) -> (error out=w200:errorcluster)  [unwired: 1 in, 2 out]
              }
            }
          }
          frame "Hidden", "Hide" {
            w201 = T7."Hidden" ("State")
            n73 = property class="VI"(reference=w207, error in=w206) -> (reference out=w204:refnum<vi>, error out=w205:errorcluster, "FP.State"=w203:T7)
            n74 = Not Equal?(x=w203, y=w201) -> (x != y?=w202:bool)
            n75 = case shown="True" w202 {
              tunnel: [w212 w213] -> w208
              tunnel: w205 -> [w211 w213]
              tunnel: w204 -> [w210 _]
              tunnel: w201 -> [w209 _]
              frame True {
                n76 = invoke class="VI" method="FP.Open"(reference=w210, error in=w211, "State"=w209) -> (error out=w212:errorcluster)  [unwired: 2 in, 4 out]
              }
              frame False {
              }
            }
          }
          frame "Minimize", "Minimized" {
            w214 = T7."Minimized" ("State")
            n77 = property class="VI"(reference=w220, error in=w219) -> (reference out=w217:refnum<vi>, error out=w218:errorcluster, "FP.State"=w216:T7)
            n78 = Not Equal?(x=w216, y=w214) -> (x != y?=w215:bool)
            n79 = case shown="True" w215 {
              tunnel: [w225 w226] -> w221
              tunnel: w218 -> [w224 w226]
              tunnel: w217 -> [w223 _]
              tunnel: w214 -> [w222 _]
              frame True {
                n80 = invoke class="VI" method="FP.Open"(reference=w223, error in=w224, "State"=w222) -> (error out=w225:errorcluster)  [unwired: 2 in, 4 out]
              }
              frame False {
              }
            }
          }
          frame "Maximize", "Maximized" {
            w227 = T7."Maximized" ("State")
            n81 = property class="VI"(reference=w233, error in=w232) -> (reference out=w230:refnum<vi>, error out=w231:errorcluster, "FP.State"=w229:T7)
            n82 = Not Equal?(x=w229, y=w227) -> (x != y?=w228:bool)
            n83 = case shown="True" w228 {
              tunnel: [w238 w239] -> w234
              tunnel: w231 -> [w237 w239]
              tunnel: w230 -> [w236 _]
              tunnel: w227 -> [w235 _]
              frame True {
                n84 = invoke class="VI" method="FP.Open"(reference=w236, error in=w237, "State"=w235) -> (error out=w238:errorcluster)  [unwired: 2 in, 4 out]
              }
              frame False {
              }
            }
          }
        }
        n85 = call <vilib>:"Add State(s) to Queue__JKI_lib_State_Machine.vi"("State(s) in (\"\")"=w174) -> ("States Out"=w173:string)  [unwired: 14 in]
      }
      frame "---------- Macro ----------" {
        # "Do not put any code in this frame.\n(It is a separator no-op. You can make a copy of this frame to create a new Macro frame)"
        n86 = call <vilib>:"Add State(s) to Queue__JKI_lib_State_Machine.vi"("State(s) in (\"\")"=w243) -> ("States Out"=w242:string)  [unwired: 14 in]
      }
      frame "Macro: Initialize" {
        w244 = "Data: Initialize\nInitialize Core Data\nControl: Initialize\nPSU: Output >> Off\nArduino: Mode >> Heat\nUI: Initialize\nUI: Front Panel State >> Open"  # Data: Initialize Initialize Core Data Control: Initialize PSU: Output >> Off Arduino: Mode >> Heat UI: Initialize UI: Front Panel State >> Open
        # "Initialization Macro\n(This is called once, when the VI starts)"
        n87 = call <vilib>:"Add State(s) to Queue__JKI_lib_State_Machine.vi"("State(s) in Front (\"\")"=w244, "State(s) in (\"\")"=w248) -> ("States Out"=w247:string)  [unwired: 13 in]
      }
      frame "Macro: Exit" {
        # "Exit Macro\n(This is called once, when the VI exits)"
        n88 = Unbundle By Name(w255) -> ("Core.Close Panel on Exit?"=w254:bool)
        n89 = Select(t="UI: Front Panel State >> Close", s=w254, f="") -> (s? t:f=w251:string)
        n90 = call <vilib>:"Add State(s) to Queue__JKI_lib_State_Machine.vi"("State(s) in (\"\")"=w251, "State(s) at Back (\"\")"="Data: Cleanup\nExit") -> ("States Out"=w249:string)  [unwired: 13 in]
        n91 = call <vilib>:"Add State(s) to Queue__JKI_lib_State_Machine.vi"("State(s) in Front (\"\")"=w249, "State(s) in (\"\")"=w258) -> ("States Out"=w257:string)  [unwired: 13 in]
      }
      frame "---------- Control ----------" {
        # "Template Separator\n(You can make a copy of, or modify, this frame)"
        n92 = call <vilib>:"Add State(s) to Queue__JKI_lib_State_Machine.vi"("State(s) in (\"\")"=w262) -> ("States Out"=w261:string)  [unwired: 14 in]
      }
      frame "Control: Initialize" {
        # "Your code here.\n(You can make a copy of, or modify, this frame)"
        n93 = Unbundle By Name(w274) -> ("Connections.cDAQ.Connected"=w272:bool, "Connections.PSU.Connected"=w270:bool, "Data Acquisition.Active"=w273:bool, "Connections.cDAQ.Active"=w269:bool)
        n94 = Not(x=w273) -> (.not. x?=w271:bool)
        n95 = Not(x=w269) -> (.not. x?=w268:bool)
        n96 = Compound Arithmetic op=AND(w272, w270, w271, w268) -> (w266:bool)
        n97 = Select(t="Control: Enable", s=w266, f="Control: Disable") -> (s? t:f=w265:string)
        n98 = Bundle By Name(cluster=w275, "Ready"=w266) -> (w267:T9)
        n99 = call <vilib>:"Add State(s) to Queue__JKI_lib_State_Machine.vi"("State(s) in Front (\"\")"=w265, "State(s) in (\"\")"=w278) -> ("States Out"=w277:string)  [unwired: 13 in]
      }
      frame "Control: Enable" {
        w279 = T6."Enabled" ("Disabled")
        # "Initialize the User Interface, here.\n(this is called automatically, by the Macro: Init)"
        n100 = property on="Start" class="Bool (strict)"("Colors [4]"=cluster{u32, u32}[] [{1985280, 12369084}, {4367360, 4367360}, {8388608, 16711681}, {1985280, 1985280}, {1985280, 4367360}, {8388608, 16711681}], "Strings [4]"=string[] ["Ready", "Active", "Stop", "Start"], "DisabledEnum"=w279) -> ()  [unwired: 2 in, 2 out]
        n101 = property on="Intensisty" class="Slide (strict)"("DisabledEnum"=w279) -> ()  [unwired: 2 in, 2 out]
        n102 = property on="Cool/Heat" class="Enum (strict)"("DisabledEnum"=w279) -> ()  [unwired: 2 in, 2 out]
        n103 = property on="Manual" class="WFChart (strict)"("DisabledEnum"=w279) -> ()  [unwired: 2 in, 2 out]
        n104 = property on="Intensisty" class="Slide (strict)"("DisabledEnum"=w279) -> ()  [unwired: 2 in, 2 out]
        n105 = call <vilib>:"Add State(s) to Queue__JKI_lib_State_Machine.vi"("State(s) in Front (\"\")"="UI: Status >> System Ready" ("State(s) in Front (\"\")"), "State(s) in (\"\")"=w286) -> ("States Out"=w285:string)  [unwired: 13 in]
      }
      frame "Control: Done" {
        # "Initialize the User Interface, here.\n(this is called automatically, by the Macro: Init)"
        n106 = local write "Start"(FALSE ("Key Focus")) -> ()
        n107 = property on="Start" class="Bool (strict)"("Colors [4]"=cluster{u32, u32}[] [{1985280, 12369084}, {4367360, 4367360}, {8388608, 16711681}, {1985280, 1985280}, {1985280, 4367360}, {8388608, 16711681}], "Strings [4]"=string[] ["Done", "Active", "Stop", "Start"]) -> ()  [unwired: 2 in, 2 out]
        n108 = One Button Dialog(message="Target temperature reached.") -> ()  [unwired: 1 in, 1 out]
        n109 = call <vilib>:"Add State(s) to Queue__JKI_lib_State_Machine.vi"("State(s) in Front (\"\")"="PSU: Output >> OFF\nUI: Status >> Temperature Reached" ("State(s) in Front (\"\")"), "State(s) in (\"\")"=w295) -> ("States Out"=w294:string)  [unwired: 13 in]
      }
      frame "Control: Disable" {
        w296 = T6."Disabled and Grayed Out" ("Disabled")
        # "Initialize the User Interface, here.\n(this is called automatically, by the Macro: Init)"
        n110 = property on="Start" class="Bool (strict)"("Colors [4]"=cluster{u32, u32}[] [{8388608, 8388608}, {8388608, 8388608}, {8388608, 8388608}, {8388608, 8388608}, {8388608, 8388608}, {16711681, 16711680}], "Strings [4]"=string[] ["Error", "Error", "Error", "Error"], "DisabledEnum"=w296) -> ()  [unwired: 2 in, 2 out]
        n111 = property on="Intensisty" class="Slide (strict)"("DisabledEnum"=w296) -> ()  [unwired: 2 in, 2 out]
        n112 = property on="Manual" class="WFChart (strict)"("DisabledEnum"=w296) -> ()  [unwired: 2 in, 2 out]
        n113 = property on="Intensisty" class="Slide (strict)"("DisabledEnum"=w296) -> ()  [unwired: 2 in, 2 out]
        n114 = property on="Cool/Heat" class="Enum (strict)"("DisabledEnum"=w296) -> ()  [unwired: 2 in, 2 out]
        n115 = Unbundle By Name(w310) -> ("Connections.PSU.Connected"=w309:bool, "Connections.cDAQ.Connected"=w308:bool, "Data Acquisition.Active"=w307:bool)
        n116 = Select(t="", s=w309, f="UI: Status >> PSU Connection Error") -> (s? t:f=w300:string)
        n117 = Select(t="", s=w308, f="UI: Status >> cDAQ Connection Error") -> (s? t:f=w299:string)
        n118 = Select(t="UI: Status >> Error! Data Acquisition Active" ("f"), s=w307, f="") -> (s? t:f=w298:string)
        n119 = call <vilib>:"Add State(s) to Queue__JKI_lib_State_Machine.vi"("State(s) in Front (\"\")"=w300, "State(s) in (\"\")"=w299, "State(s) at Back (\"\")"=w298) -> ("States Out"=w297:string)  [unwired: 12 in]
        n120 = call <vilib>:"Add State(s) to Queue__JKI_lib_State_Machine.vi"("State(s) in Front (\"\")"=w297, "State(s) in (\"\")"=w316) -> ("States Out"=w315:string)  [unwired: 13 in]
      }
      frame "Control: Start" {
        # "Your code here.\n(You can make a copy of, or modify, this frame)"
        n121 = Unbundle By Name(w319) -> ("Ready"=w318:bool)
        n122 = Bundle By Name(cluster=w319, "Active"=w318) -> (w320:T9)
        n123 = call <vilib>:"Add State(s) to Queue__JKI_lib_State_Machine.vi"("State(s) in Front (\"\")"="PSU: Output >> True" ("State(s) in Front (\"\")"), "State(s) in (\"\")"=w323) -> ("States Out"=w322:string)  [unwired: 13 in]
      }
      frame "---------- PSU ----------" {
        # "Template Separator\n(You can make a copy of, or modify, this frame)"
        n124 = call <vilib>:"Add State(s) to Queue__JKI_lib_State_Machine.vi"("State(s) in (\"\")"=w327) -> ("States Out"=w326:string)  [unwired: 14 in]
      }
      frame "PSU: Output" {
        # "Template Separator\n(You can make a copy of, or modify, this frame)"
        n125 = Unbundle By Name(w331) -> ("Connections.PSU.Connected"=w332:bool)
        n126 = case shown="True" w332 {
          tunnel: w331 -> [_ w340]
          tunnel: w330 -> [_ w339]
          tunnel: w329 -> [w336 w338]
          tunnel: [w336 w337] -> w328
          frame False {
          }
          frame True {
            n127 = call "PSU_State.vi"("error in (no error)"=w338, "Arguments"=w339, "DataCluster"=w340) -> ("error out"=w337:errorcluster)  [unwired: 6 in, 2 out]
          }
        }
        n128 = call <vilib>:"Add State(s) to Queue__JKI_lib_State_Machine.vi"("State(s) in (\"\")"=w335) -> ("States Out"=w334:string)  [unwired: 14 in]
      }
      frame "Arduino: Mode" {
        # "Template Separator\n(You can make a copy of, or modify, this frame)"
        n129 = call "Arduino_Mode.vi"("Arguments"=w342, "input cluster"=w343) -> ()  [unwired: 7 in, 3 out]
        n130 = call <vilib>:"Add State(s) to Queue__JKI_lib_State_Machine.vi"("State(s) in (\"\")"=w346) -> ("States Out"=w345:string)  [unwired: 14 in]
      }
    }
    n131 = call <extravilib>:"Write.vi"("element"=w17) -> ("channel"=w10:T11)  [unwired: 1 out]
    n132 = call <extravilib>:"Write.vi"("element"=w16) -> ("channel"=w9:T12)  [unwired: 1 out]
  }
  n133 = while {
    tunnel: [w354] -> w6
    tunnel: "error in" -> [w353]
    tunnel: [w352] -> w3
    tunnel: w1 -> [w347]
    tunnel: w2 -> [w349]
    tunnel: "DataCluster" -> [w355]
    stop <- w348 stop-if-true
    n134 = call <extravilib>:"Read.vi"("channel"=w347) -> ("element"=w351:T9)  [unwired: 1 in, 1 out]
    n135 = call <extravilib>:"Read.vi"("channel"=w349) -> ("element"=w348:bool)  [unwired: 1 in, 1 out]
    n136 = Unbundle By Name(w351) -> ("Active"=w350:bool)
    n137 = case shown="True" w350 {
      tunnel: w355 -> [_ w364]
      tunnel: [w356 w363] -> w354
      tunnel: w353 -> [w356 w361]
      tunnel: [_ w360] -> w352
      tunnel: w349 -> [_ w359]
      tunnel: w347 -> [_ w358]
      frame False {
        n138 = Wait (ms)(milliseconds to wait=u32 100) -> ()  [unwired: 1 out]
      }
      frame True {
        n139 = call "SampleRate_Convert.vi"("DataCluster"=w364) -> ("Sample dt (ms)"=w362:i64)  [unwired: 1 out]
        n140 = node-c288(w362, w361) -> (w366:T13)
        n141 = timed-loop {
          tunnel: w359 -> [w383]
          timing: w366 -> [_]
          timing-out: [_] -> w365
          tunnel: [w373] -> w360
          tunnel: w358 -> [w371]
          tunnel: w364 -> [w379]
          stop <- w384 stop-if-true
          n142 = node-c288() -> (w378:errorcluster)  [unwired: 1 in]
          n143 = call <extravilib>:"Read.vi"("channel"=w371) -> ("element"=w370:T9)  [unwired: 1 in, 1 out]
          n144 = Unbundle By Name(w370) -> ("Cool/Heat"=w367:enum32{"Cool", "Heat"}, "Active"=w368:bool)
          n145 = call <extravilib>:"Read.vi"("channel"=w383) -> ("element"=w382:bool)  [unwired: 1 in, 1 out]
          n146 = Not(x=w368) -> (.not. x?=w369:bool)
          n147 = Or(x=w369, y=w382) -> (x .or. y?=w372:bool)
          n148 = call "Manual_Cool_Control.vi"("Intensity"="Intensisty", "Cool/Heat"=w367, "DataCluster"=w379) -> ("Output %"=w375:i32, "DataCluster out"=w376:T1, "Temps"=→"Manual":waveform(dbl)[], "Reached Temp"=w374:bool)  [unwired: 5 in]
          n149 = call <extravilib>:"Write.vi"("element"=w374) -> ("channel"=w373:T16)  [unwired: 8 in, 2 out]
          n150 = call "PSU_Output.vi"("error in (no error)"=w378, "Output %"=w375, "DataCluster in"=w376) -> ("error out"=w377:errorcluster)  [unwired: 6 in, 2 out]
          n151 = Or(x=w377, y=w372) -> (x .or. y?=w384:bool)
          n152 = node-c288(w377) -> ()  [unwired: 1 out]
        }
        n153 = node-c288(w365) -> (w363:errorcluster)
      }
    }
  }
  "error out" <- w6
